vi "Read signal std.vi"(8 "error in (no error)":errorcluster, 11 "processingTA in":refnum<class "processingTA.lvclass">) -> (0 "error out":errorcluster, 2 "signal std":dbl[](array[numeric]), 3 "processingTA out":refnum<class "processingTA.lvclass">)   [LabVIEW 2019, in "processingTA.lvlib" / "processingTA.lvclass"]
uses:
  processingTA.lvclass
  processingTA.lvclass/processingTA.ctl
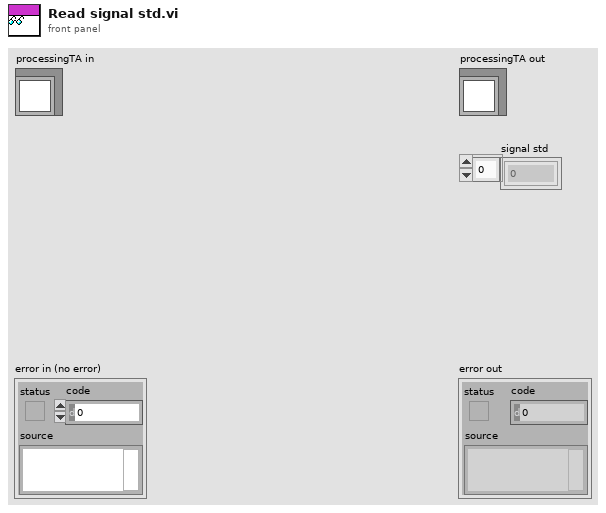
[diagram p1: front panel]
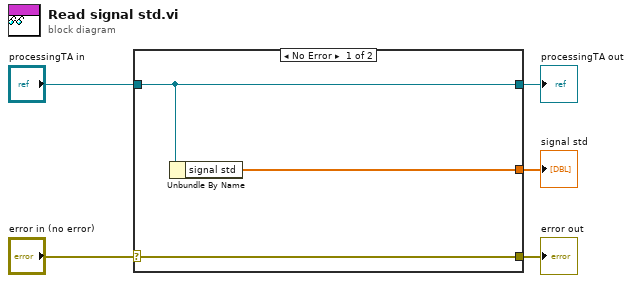
[diagram p0: block diagram]
diagram:
  n1 = case shown="No Error" "error in (no error)" {
    selector: "error in (no error)" -> [w8 w9]
    tunnel: [w8 w9] -> w4
    tunnel: [w7 w10] -> w2
    tunnel: "processingTA in" -> [w7 w10]
    tunnel: [w6 _] -> w1
    frame No Error {
      n2 = Unbundle By Name(w7) -> ("signal std"=w6:dbl[])
    }
    frame Error {
    }
  }
  "error out" <- w4
  "processingTA out" <- w2
  "signal std" <- w1
